vi "T7MOD_Read_UINT16_Register.vi"(8 "error in":errorcluster, 9 "LabJack UINT16 Register":i32=55110, 10 "Remote Port":u16=502, 11 "Remote IP Address":string="192.168.1.15") -> (0 "error out":errorcluster, 1 "Read At":timestamp, 2 "Raw Data Read":u16[](array[numeric]), 3 "Read UINT16":u16)   [LabVIEW 2015]
uses:
  Serial Link Layer/NI_Modbus_Cleaned/NI Modbus121Clean.llb/MB Ethernet Master Query Read Input Registers (poly).vi
panel:
  # "Output"
  # "TCP Parameters"
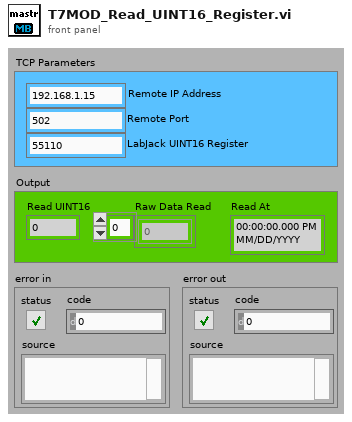
[diagram p1: front panel]
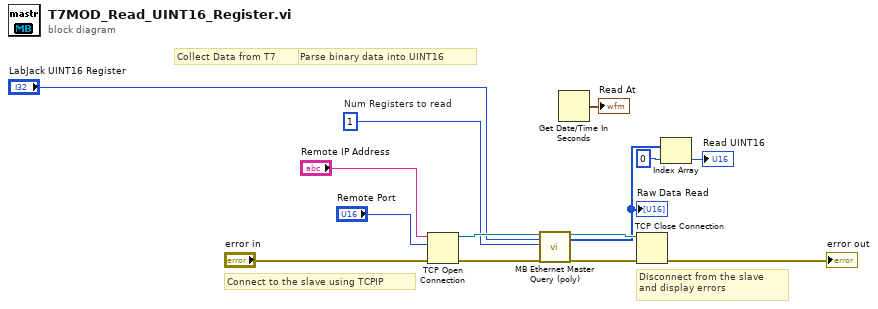
[diagram p0: block diagram]
diagram:
  w7 = 1  # Num Registers to read
  # "Parse binary data into UINT16"
  # "Collect Data from T7"
  # "Disconnect from the slave\nand display errors"
  # "Connect to the slave using TCPIP"
  n1 = TCP Open Connection(address="Remote IP Address", remote port or service name="Remote Port", error in (no error)="error in") -> (connection ID=w12:refnum<k5>, error out=w11:errorcluster)  [unwired: 2 in]
  n2 = call-poly "MB Ethernet Master Query (poly).vi"("TCP Connection Refnum in"=w12, "Starting Address"="LabJack UINT16 Register", "Quantity"=w7, "error in"=w11) -> ("TCP Connection Refnum (dup)"=w9:refnum<k5>, "Input Registers"=w4:u16[], "error out"=w10:errorcluster)  [unwired: 12 in, 1 out]
  "Raw Data Read" <- w4
  n3 = Get Date/Time In Seconds() -> (seconds since 1Jan1904=→"Read At":timestamp)
  n4 = TCP Close Connection(connection ID=w9, error in (no error)=w10) -> (error out=→"error out":errorcluster)  [unwired: 2 out]
  n5 = Index Array(array=w4, index=0) -> (element=→"Read UINT16":u16)
